vi "AddDataListener.vi"(8 "error in (no error)":errorcluster, 9 "Listener In":refnum<class "Message Enqueuer.lvclass">, 10 "Label":string, 11 "GRMActor in":refnum<class "GenericController.lvclass">) -> (0 "error out":errorcluster, 3 "GRMActor out":refnum<class "GenericController.lvclass">)   [LabVIEW 2020, in "GenericController.lvlib" / "GenericController.lvclass"]
uses:
  GenericController.lvclass
  <vilib>/ActorFramework/Message Enqueuer/Message Enqueuer.lvclass
  GenericController.lvclass/GenericController.ctl
panel:
  out "key already included?":bool
  out "value unchanged?":bool
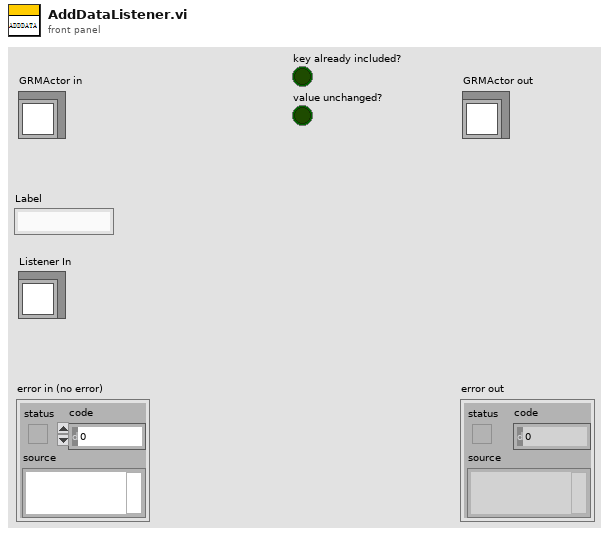
[diagram p1: front panel]
types:
  T1 = map{string, refnum<class "Message Enqueuer.lvclass">}
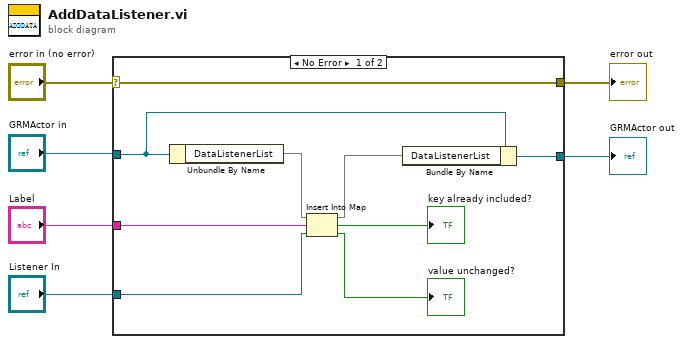
[diagram p0: block diagram]
diagram:
  n1 = case shown="No Error" "error in (no error)" {
    selector: "error in (no error)" -> [w15 w17]
    tunnel: [w15 w17] -> w2
    tunnel: [w14 w16] -> w1
    tunnel: "GRMActor in" -> [w13 w16]
    tunnel: "Label" -> [w8 _]
    tunnel: "Listener In" -> [w7 _]
    frame No Error {
      n2 = Unbundle By Name(w13) -> ("DataListenerList"=w12:T1)
      n3 = Insert Into Map(map in=w12, key=w8, value=w7) -> (map out=w11:T1, key already included?=→"key already included?":bool, value unchanged?=→"value unchanged?":bool)
      n4 = Bundle By Name(cluster=w13, "DataListenerList"=w11) -> (w14:refnum<class "GenericController.lvclass">)
    }
    frame Error {
    }
  }
  "error out" <- w2
  "GRMActor out" <- w1
